vi "GetAllClass.vi"(8 "error in (no error)":errorcluster) -> (0 "error out":errorcluster, 2 "Not owned (outside .lvlib)":path[](array[path]), 3 "Owned class (in .lvlib)":path[](array[path]), 5 "Lvclass paths":path[](array[path]))   [LabVIEW 2019, in "Hawkeye.lvlib"]
uses:
  Hawkeye.lvlib
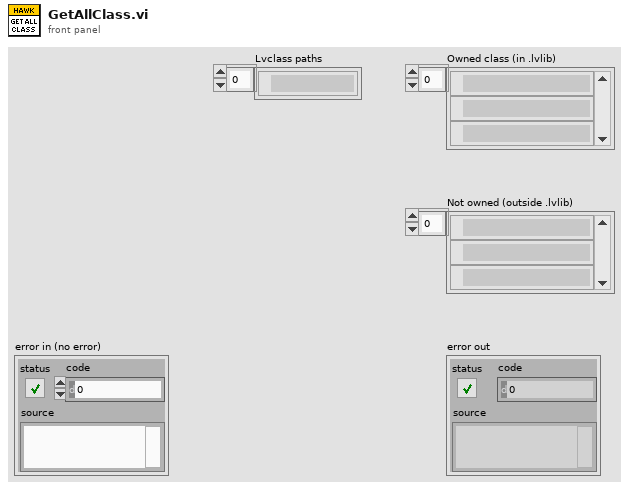
[diagram p1: front panel]
types:
  T1 = typedef "Hawkeye.lvlib/HawkeyePathConfigs.ctl" = cluster{"GlobalIncludePaths":path[], "GlobalExcludePaths":path[], "BuildSpecsIncludePaths":path[], "ActualDepsIncludePaths":path[], "WorkspacePath":path, "SourceFolderPaths":path[], "ChangedFilesLogpaths":map{string, path}}
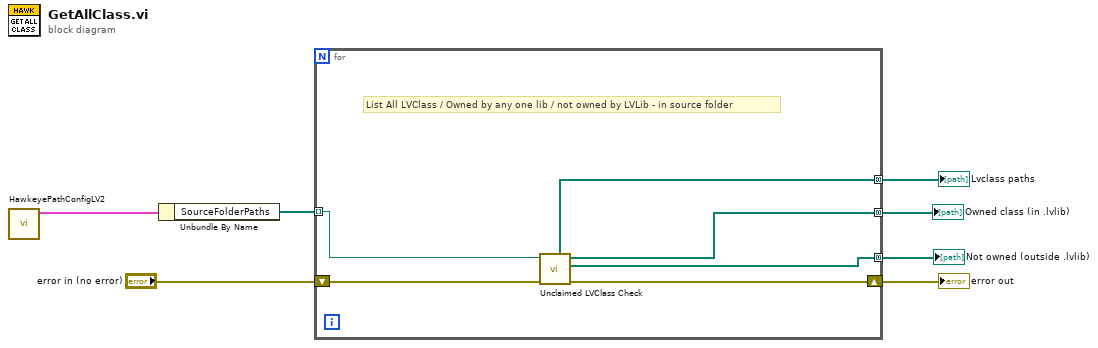
[diagram p0: block diagram]
diagram:
  n1 = call "HawkeyePathConfigLV2.vi"() -> ("Hawkeye Path Config Out"=w3:T1)  [unwired: 11 in]
  n2 = Unbundle By Name(w3) -> ("SourceFolderPaths"=w6:path[])
  n3 = for {
    tunnel: [w11] -> w4 mode=concatenating
    shift-right: [w13] -> w5
    shift-left: "error in (no error)" -> [w8]
    tunnel: w6 -> [w12] mode=indexing
    tunnel: [w10] -> w2 mode=concatenating
    tunnel: [w9] -> w1 mode=concatenating
    # "List All LVClass / Owned by any one lib / not owned by LVLib - in source folder"
    n4 = call "Unclaimed LVClass Check.vi"("error in (no error)"=w8, "Source Folder Path"=w12) -> ("error out"=w13:errorcluster, "Not owned (outside .lvlib)"=w9:path[], "Owned class (in .lvlib)"=w10:path[], "All Class Paths"=w11:path[])  [unwired: 6 in]
  }
  "error out" <- w5
  "Lvclass paths" <- w4
  "Owned class (in .lvlib)" <- w2
  "Not owned (outside .lvlib)" <- w1
